vi "Check Status.vi"(8 "error in (no error)":errorcluster, 11 "LCD Retarder in":refnum<class "LCD Retarder.lvclass">) -> (0 "error out":errorcluster, 1 "Status":string, 2 "Ready?":bool, 3 "LCD Retarder out":refnum<class "LCD Retarder.lvclass">)   [LabVIEW 2009, in "LCD Retarder.lvclass"]
doc: "Checks if the instrument is powered on and updates its member data with the instrument's current status."
uses:
  LCD Retarder.lvclass
  Utility Classes/Readable/Readable.lvclass
  LCD Retarder.lvclass/LCD Retarder.ctl
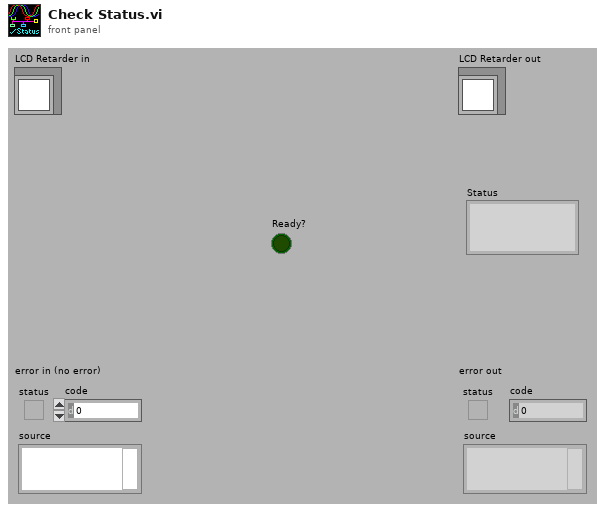
[diagram p1: front panel]
types:
  T1 = typedef "Readable.lvclass/X array.ctl" = T2[]
  T2 = typedef "Readable.lvclass/X.ctl" = dbl
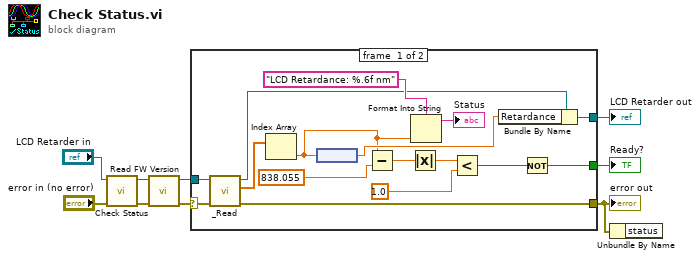
[diagram p0: block diagram]
diagram:
  n1 = call-parent "Check Status.vi"("error in (no error)"="error in (no error)", "Instrument in"="LCD Retarder in") -> ("error out"=w3:errorcluster, "Instrument out"=w6:refnum<class "LCD Retarder.lvclass">)  [unwired: 8 out]
  n2 = call "Read FW Version.vi"("errorIN"=w3, "LCD in"=w6) -> ("error out"=w2:errorcluster, "LCD out"=w5:refnum<class "LCD Retarder.lvclass">)  [unwired: 8 out]
  n3 = case shown="No Error" w2 {
    selector: w2 -> [w24 w26]
    tunnel: [w25 w26] -> w4
    tunnel: w5 -> [w23 w27]
    tunnel: [w20 w27] -> w7
    tunnel: [w13 _] -> w1
    frame #0 {
      n4 = call-dynamic "_Read.vi"("errorIN"=w24, "LCD in"=w23) -> ("errorOUT"=w25:errorcluster, "X array"=w19:T1, "LCD out"=w18:refnum<class "LCD Retarder.lvclass">)  [unwired: 7 out]
      n5 = Index Array(array=w19) -> (element=w11:T2)  [unwired: 1 in]
      n6 = node(w11) -> (w17:dbl[unit])
      n7 = Subtract(x=w11, y=838.055) -> (x-y=w16:T2)
      n8 = Absolute Value(x=w16) -> (abs(x)=w14:T2)
      n9 = Format Into String(format string="LCD Retardance: %.6f nm", w11) -> (resulting string=→"Status":string)  [unwired: 2 in, 1 out]
      n10 = Less?(x=w14, y=1.0) -> (x < y?=w15:bool)
      n11 = Bundle By Name(cluster=w18, "Retardance"=w17) -> (w20:refnum<class "LCD Retarder.lvclass">)
      n12 = Not(x=w15) -> (.not. x?=w13:bool)
    }
    frame #1 {
    }
  }
  "error out" <- w4
  "LCD Retarder out" <- w7
  "Ready?" <- w1
  n13 = Unbundle By Name(w4) -> ()  [unwired: 1 out]
